vi "4.6.（4）.vi"() -> ()   [LabVIEW 2017]
panel:
  out "和":dbl
  in  "加数2":dbl
  in  "加数1":dbl
  in  "停止":bool
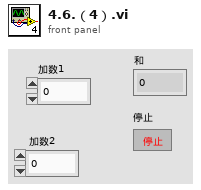
[diagram p1: front panel]
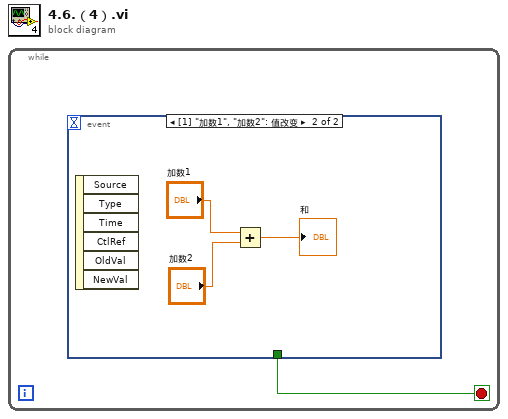
[diagram p0: block diagram]
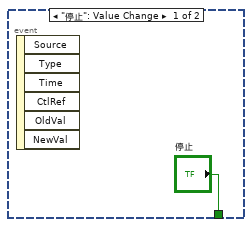
[diagram p2: hidden frame]
diagram:
  n1 = while {
    stop <- w1 stop-if-true
    n2 = event shown="[1] \"加数1\", \"加数2\": 值改变" {
      selector: _ -> [_ _]
      dyn-events: _ -> [_ _]
      timeout: _ -> [_ _]
      tunnel: ["停止" _] -> w1
      event "停止": Value Change {
        n3 = event-data() -> ()  [unwired: 1 in, 6 out]
      }
      event "加数1", "加数2": Value Change {
        n4 = event-data() -> ()  [unwired: 1 in, 6 out]
        n5 = Add(x="加数1", y="加数2") -> (x+y=→"和":dbl)
      }
    }
  }
